vi "Main_01.vi"() -> ()   [LabVIEW 2023]
panel:
  out "sum":i32
  out "Array":i32[](array[numeric])
  in  "Puzzle":string="9cbncbxclbvkmfzdnldc\njjn1drdffhs\n3six7\n38rgtnqqxtc\nrxszdkkv3j8kjhbm\n54nzzddht8ninelrkkseightseven6\n6fourmnvkgnthjtnjqkr\nnineninezsstmkone4sjnlbldcrj4eight\n3rdnfkvrx4twoqgeightqkgmn\n6mlhponeglrzrvbsseven\nfive8spgxz8\n3three2dfourfour58\n9q\ntwo45\nfive8mpkpdfiveeightfourseven\n93threefive3three92\n6jdzeightnineone1sclhzrnrjxfive\n6nseven16lbztpbbzthree8five\neight6mntljvbfrmftsffchsix4\n4twosixvnhjl\n8d\neightsevenvqvzlqxkbm6rqhsgqpnine7twonex\nseven96\nck8tv6\n2mcddqpnbxssmrc6\nzsfbkrjjqpbbone6six2\nfourone8hfrkxrr\n7ninetphdpcx\n9gcn9six4mfnjgtcdc\n6onevsevenseven4three\nldssggpknine7\ntwolltbfkhltwo892jngx\nrsh1f..."
  in  "Sample":string="1abc2\npqr3stu8vwx\na1b2c3d4e5f\ntreb7uchet"
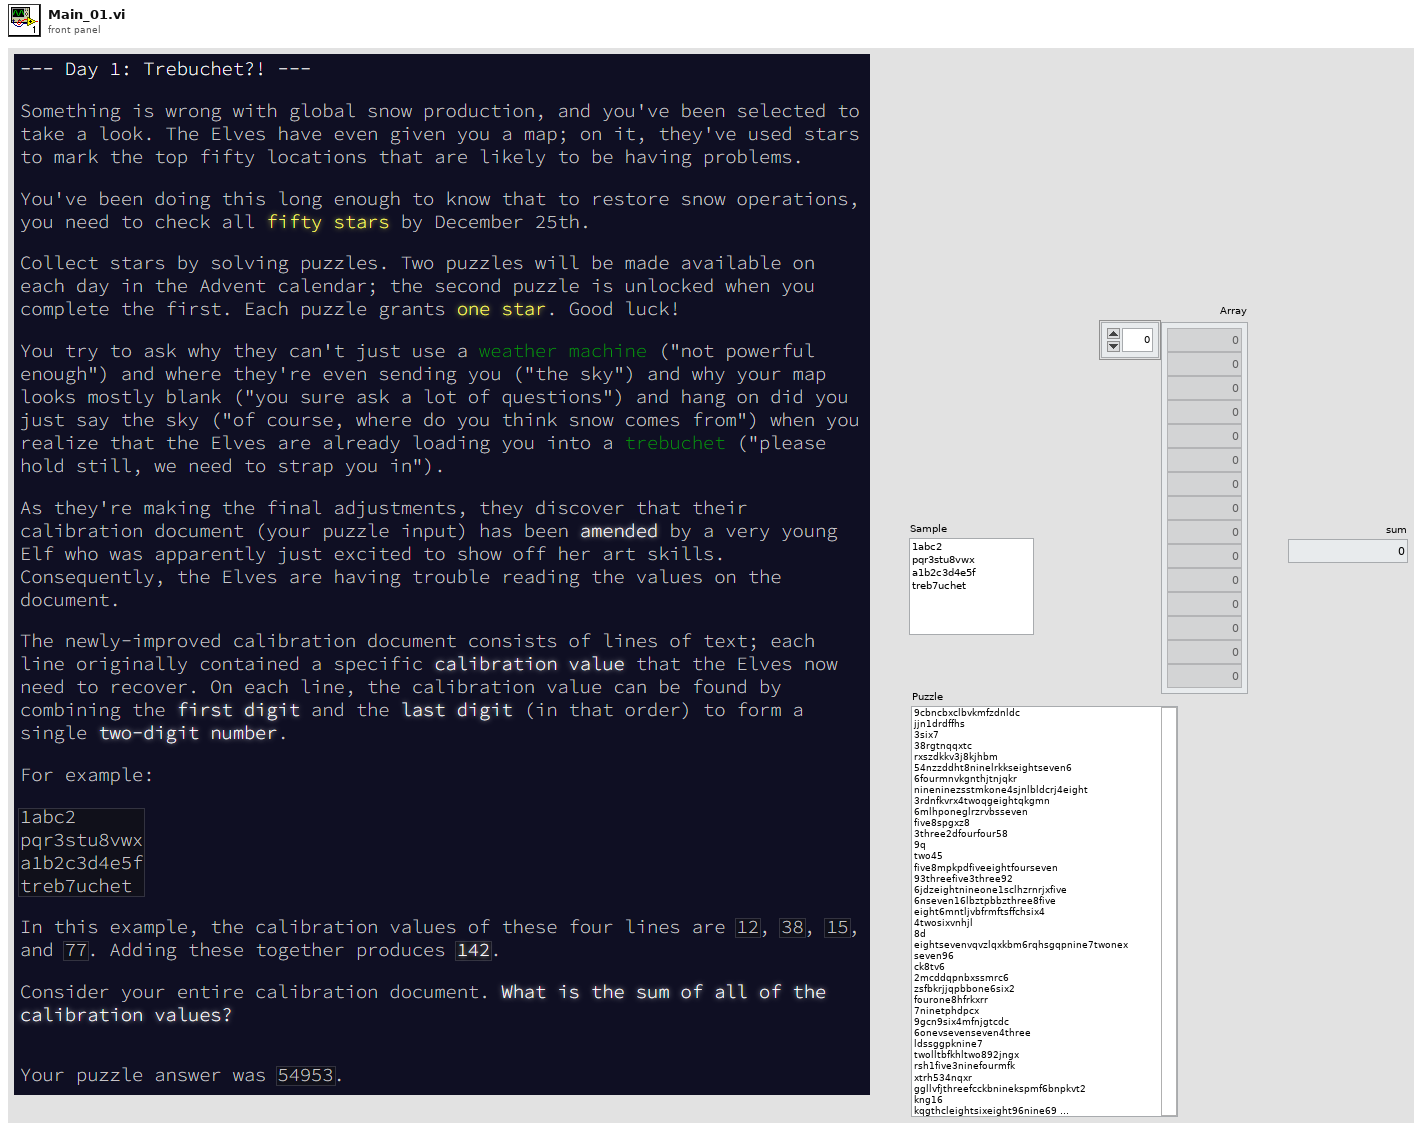
[diagram p1: front panel]
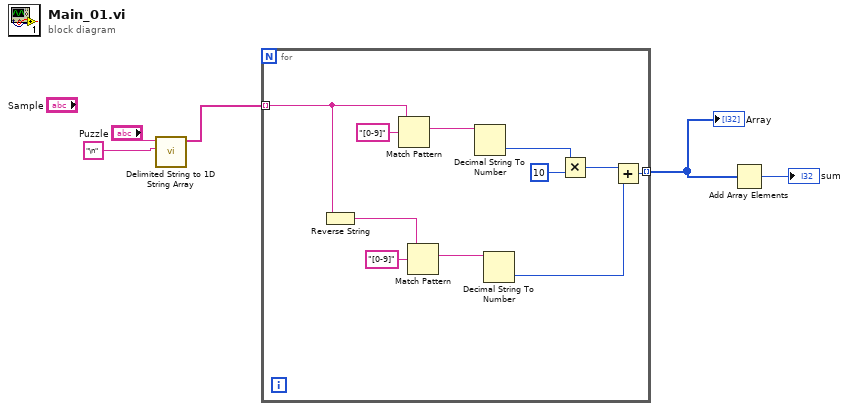
[diagram p0: block diagram]
diagram:
  n1 = call <vilib>:"Delimited String to 1D String Array.vi"("delimiter"="\n", "delimited string"="Puzzle") -> ("string array"=w4:string[])  [unwired: 9 in]
  n2 = for {
    tunnel: w4 -> [w11] mode=indexing
    tunnel: [w6] -> w3 mode=indexing
    n3 = Reverse String(1:w11) -> (0:w12:string)
    n4 = Match Pattern(string=w11, regular expression="[0-9]") -> (match substring=w15:string)  [unwired: 1 in, 3 out]
    n5 = Match Pattern(string=w12, regular expression="[0-9]") -> (match substring=w14:string)  [unwired: 1 in, 3 out]
    n6 = Decimal String To Number(string=w15) -> (number=w10:i32)  [unwired: 2 in, 1 out]
    n7 = Decimal String To Number(string=w14) -> (number=w7:i32)  [unwired: 2 in, 1 out]
    n8 = Multiply(x=w10, y=10) -> (x*y=w8:i32)
    n9 = Add(x=w8, y=w7) -> (x+y=w6:i32)
  }
  "Array" <- w3
  n10 = Add Array Elements(numeric array=w3) -> (sum=→"sum":i32)
